vi "feedback.vi"() -> ()   [LabVIEW 2014]
uses:
  <vilib>/FTP/NI_FTP.lvlib
panel:
  in  "확인 버튼":bool
  in  "닫기":bool
  in  "전송":bool
  in  "Subject":string="\u001b¼”²¬ÀŒ·" caption="제목"
  in  "Message":string="제목을 입력해 주세요." caption="메시지"
  # "TºÜÂÀÉÈ¡Á"
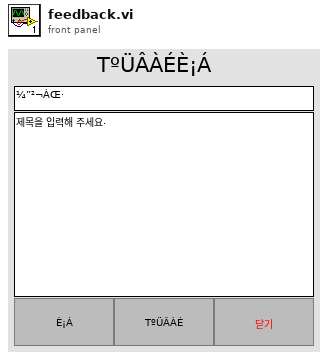
[diagram p1: front panel]
types:
  T1 = typedef "NI_FTP.lvlib/FTP Session.ctl" = refnum<k5>
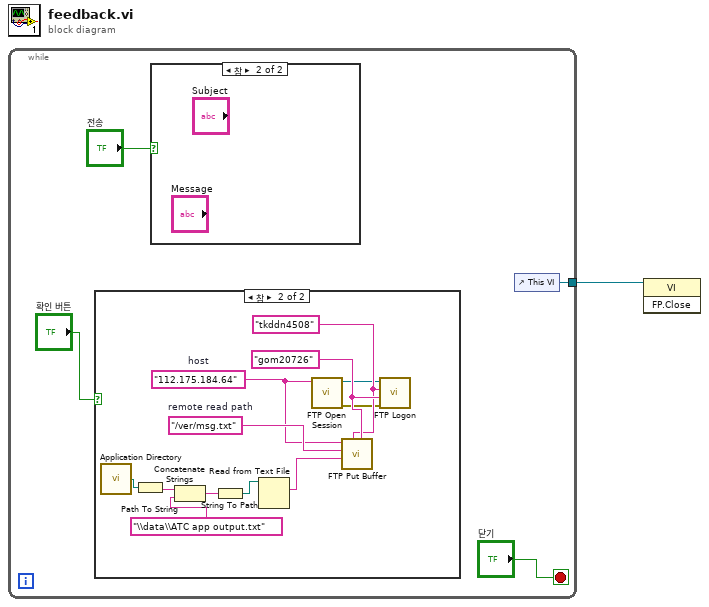
[diagram p0: block diagram]
diagram:
  n1 = while {
    tunnel: [w5] -> w1
    stop <- "닫기" stop-if-true
    n2 = case shown="참" "확인 버튼" {
      frame False {
      }
      frame True {
        w15 = "gom20726"
        w14 = "tkddn4508"
        w17 = "/ver/msg.txt"  # remote read path
        w16 = "112.175.184.64"  # host
        n3 = call <vilib>:"Application Directory.vi"() -> ("Application Directory"=w11:path)
        n4 = Path To String(path=w11) -> (string=w9:string)
        n5 = Concatenate Strings(w9, "\\data\\ATC app output.txt" ("문자열")) -> (w8:string)
        n6 = String To Path(string=w8) -> (path=w7:path)
        n7 = Read from Text File(file (use dialog)=w7) -> (text=w6:string)  [unwired: 3 in, 3 out]
        n8 = call <vilib>:"FTP Open Session.vi"("address"=w16) -> ("error out"=w13:errorcluster, "ftp session"=w12:T1)  [unwired: 7 in, 2 out]
        n9 = call <vilib>:"FTP Put Buffer.vi"("password"=w15, "user"=w14, "data"=w6, "remote path"=w17, "host"=w16) -> ()  [unwired: 5 in, 2 out]
        n10 = call <vilib>:"FTP Logon.vi"("error in (no error)"=w13, "password"=w15, "user"=w14, "ftp session"=w12) -> ()  [unwired: 4 in, 4 out]
      }
    }
    n11 = case shown="참" "전송" {
      frame False {
      }
      frame True {
      }
    }
    n12 = control-ref of="This VI"() -> (w5:refnum<vi>)
  }
  n13 = invoke class="VI" method="FP.Close"(reference=w1) -> ()  [unwired: 2 in, 3 out]
